vi "GetDataTrFreq.vi"(8 "错误输入（无错误）":errorcluster) -> (0 "错误输出":errorcluster, 3 "返回值":sgl)   [LabVIEW 2018]
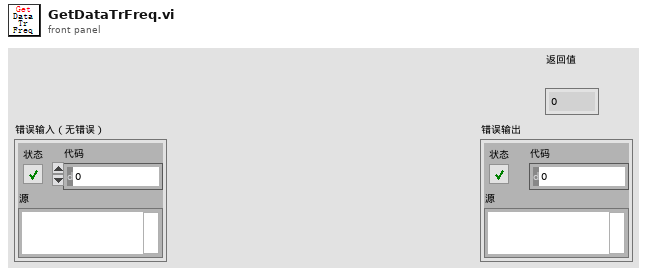
[diagram p1: front panel]
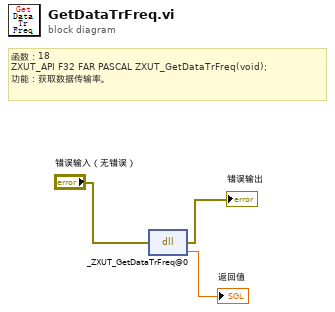
[diagram p0: block diagram]
diagram:
  # "函数：18\nZXUT_API F32\tFAR PASCAL ZXUT_GetDataTrFreq(void);\n功能：获取数据传输率。"
  n1 = dll-call lib="PTH2Rabs E软件项目超声超声子VI函数VI\tTCG处理ZXUTConfigMgr.dll" fn="_ZXUT_GetDataTrFreq@0"(error in="错误输入（无错误）") -> (error out=→"错误输出":errorcluster, "返回值"=→"返回值":sgl)  [unwired: 2 in, 1 out]
